vi "Get_Device_NameIP.vi"(8 "error in (no error)":errorcluster, 11 "Device in":refnum<class "DAQ_Device.lvclass">) -> (0 "error out":errorcluster, 1 "Device Name":string, 2 "Device Address":string, 3 "Device out":refnum<class "DAQ_Device.lvclass">, 4 "IO Channels":T1, 5 "Unit ID":u8)   [LabVIEW 2023, in "DAQ_Device.lvclass"]
uses:
  DAQ_Device.lvclass
  DAQ Device_IO ChannelsData.ctl
  DAQ_Device.lvclass/DAQ_Device.ctl
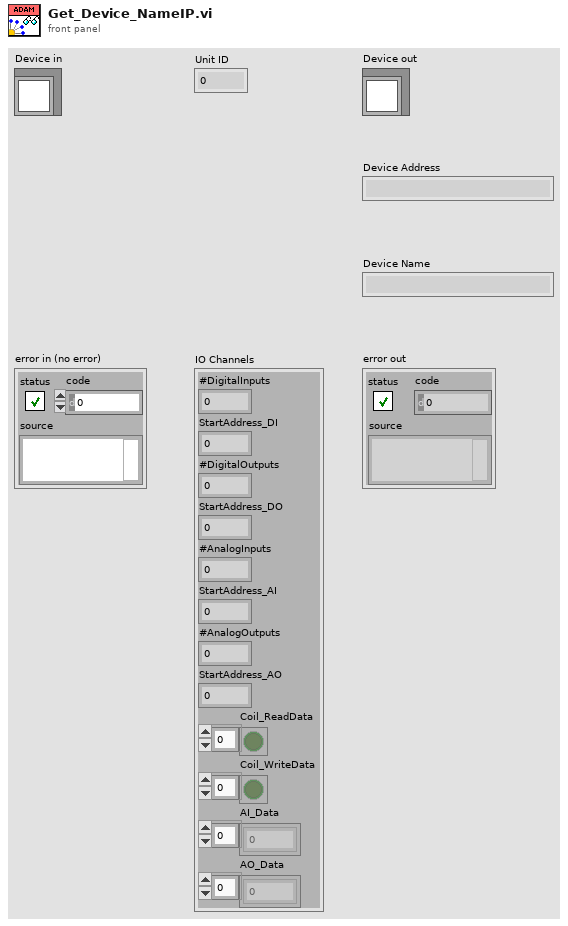
[diagram p1: front panel]
types:
  T1 = typedef "DAQ Device_IO ChannelsData.ctl" = cluster{"#DigitalInputs":u16, "StartAddress_DI":u16, "#DigitalOutputs":u16, "StartAddress_DO":u16, "#AnalogInputs":u16, "StartAddress_AI":u16, "#AnalogOutputs":u16, "StartAddress_AO":u16, "Coil_ReadData":bool[], "Coil_WriteData":bool[], "AI_Data":u16[], "AO_Data":u16[]}
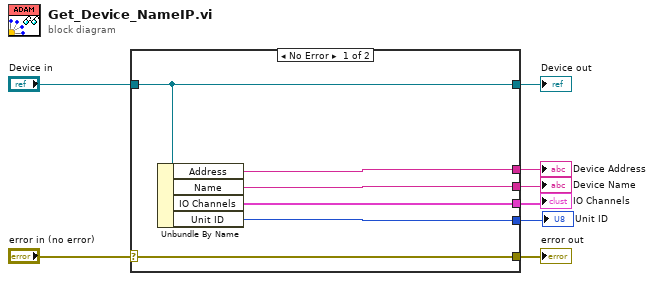
[diagram p0: block diagram]
diagram:
  n1 = case shown="No Error" "error in (no error)" {
    selector: "error in (no error)" -> [w14 w15]
    tunnel: [w14 w15] -> w7
    tunnel: [w13 w16] -> w5
    tunnel: "Device in" -> [w13 w16]
    tunnel: [w12 _] -> w4
    tunnel: [w11 _] -> w3
    tunnel: [w10 _] -> w2
    tunnel: [w9 _] -> w1
    frame No Error {
      n2 = Unbundle By Name(w13) -> ("Address"=w12:string, "Name"=w11:string, "IO Channels"=w10:T1, "Unit ID"=w9:u8)
    }
    frame Error {
    }
  }
  "error out" <- w7
  "Device out" <- w5
  "Device Address" <- w4
  "Device Name" <- w3
  "IO Channels" <- w2
  "Unit ID" <- w1
